vi "Configure Channels.vi"(8 "error in":errorcluster, 11 "HDO4000A Base CFG in":refnum<class "HDO4000A Base CFG.lvclass">) -> (0 "error out":errorcluster, 3 "HDO4000A Base CFG out":refnum<class "HDO4000A Base CFG.lvclass">)   [LabVIEW 2023, in "HDO4000A Base CFG.lvclass"]
uses:
  HDO4000A Base CFG.lvclass
  D:/git/HAL/Configuration Base/Configuration Base.lvclass
  D:/git/HAL/Scope VISA/Configuration/Scope VISA CFG.lvclass
  HAL/Scope VISA/Configuration/Scope VISA CFG.lvclass/Scope VISA CFG.ctl
  HAL/Configuration Base/Configuration Base.lvclass/Configuration Base.ctl
  1880163a-4361-407a-b3a4-4a21bf3de2cd.vi
  95c443c2-3777-477c-973f-d948cfa8a8a4.vi
  0a1f02e3-89ee-415e-b632-0a5c4b782606.vi
  6b7b7499-5745-4b63-8d29-6fa9ae9ebfc2.vi
  0b9faeda-f93b-43a9-80fc-245254112aa6.vi
  15a4e368-5e2e-4ceb-9445-3dca4af458c7.vi
  f2f44aa7-3266-48fd-b649-b0f434fb3c1c.vi
  aee8a4b4-0c09-4a90-9b34-d1bd9b76e547.vi
  <vilib>/JDP Science/JSONtext/Find Item.vi
  <vilib>/JDP Science/JSONtext/Next JSON Value.vi
  <vilib>/JDP Science/JSONtext/String Subset.vi
  <vilib>/JDP Science/JSONtext/Parsing/Advance past next JSON Value (inlined COPY).vi
  <vilib>/JDP Science/JSONtext/Parsing/Advance past whitespace.vi
  <vilib>/JDP Science/JSONtext/Parsing/Advance past String.vi
  <vilib>/JDP Science/JSONtext/Parsing/Advance past Number.vi
  <vilib>/JDP Science/JSONtext/Parsing/Advance past Line Ending.vi
  <vilib>/JDP Science/JSONtext/Parsing/Parse Full Path or Item Name.vi
  <vilib>/JDP Science/JSONtext/Parsing/Advance past Array.vi
  <vilib>/JDP Science/JSONtext/Parsing/Advance past Object.vi
  <vilib>/JDP Science/JSONtext/support/Error Cluster From Code.vi
  <vilib>/JDP Science/JSONtext/Offset/Find Item Locations by Path.vi
  <vilib>/JDP Science/JSONtext/JSON text to Variant.vi
  <vilib>/Utility/error.llb/Error Cluster From Error Code.vi
  <vilib>/JDP Science/JSONtext/LVClass Serializer/JSONtext LVClass Serializer.lvclass
  <vilib>/ErrorRing/Error Ring.xnode
  HDO4000A Base CFG.lvclass/HDO4000A Base CFG.ctl
  <instrlib>/LeCroy Wave Series/LeCroy Wave Series.lvlib
  HAL/Scope VISA/Configuration/Scope VISA CFG.lvclass
  HAL/Configuration Base/Configuration Base.lvclass
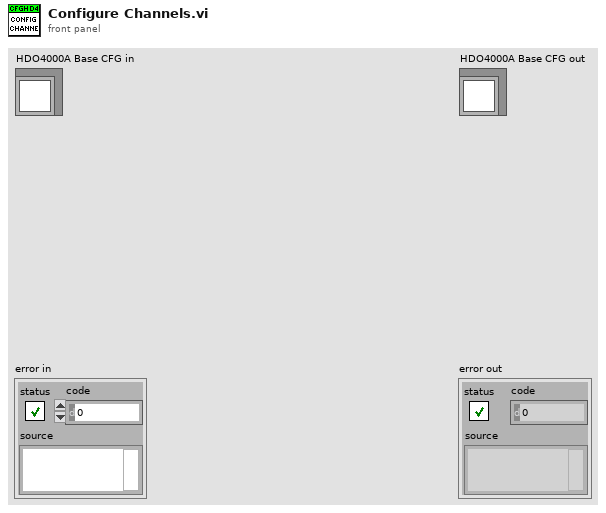
[diagram p1: front panel]
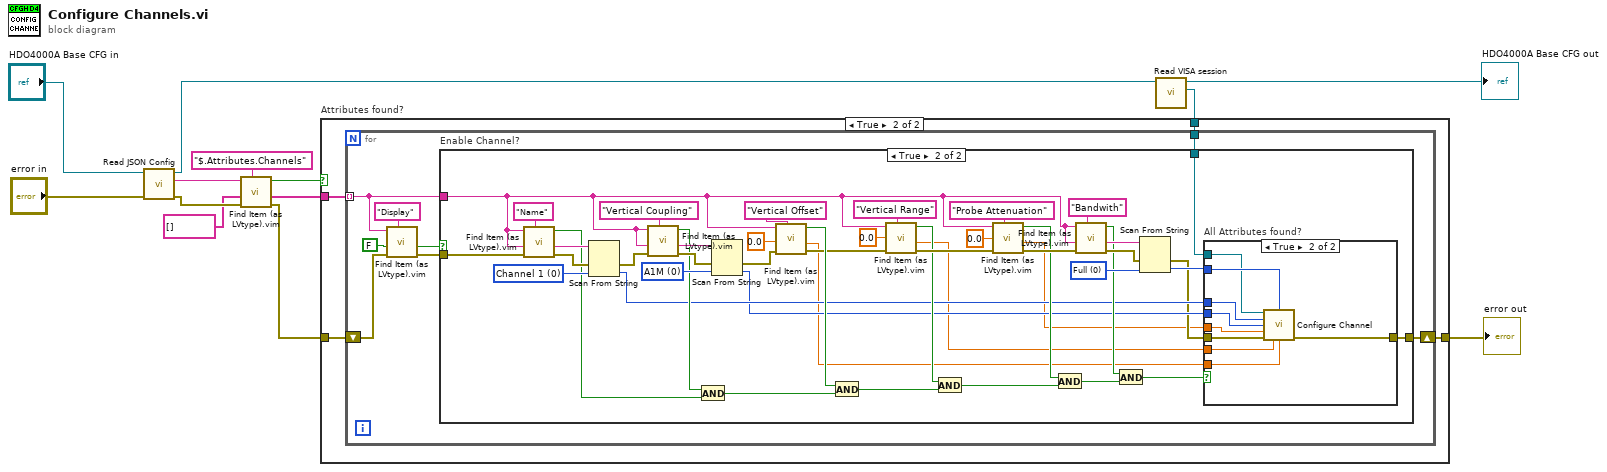
[diagram p0: block diagram]
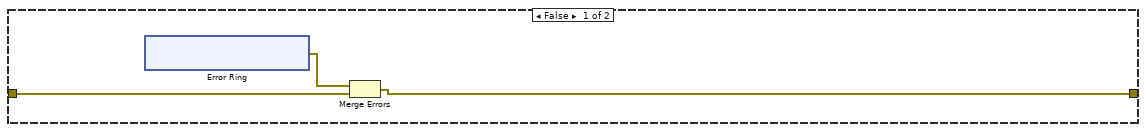
[diagram p2: hidden frame]
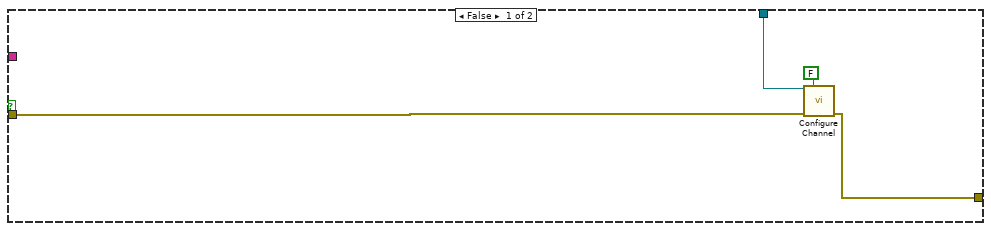
[diagram p3: hidden frame]
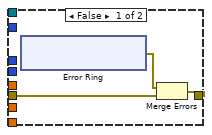
[diagram p4: hidden frame]
diagram:
  n1 = call "Read JSON Config.vi"("error in (no error)"="error in", "object in"="HDO4000A Base CFG in") -> ("error out"=w11:errorcluster, "<JSON>Config"=w8:string, "object out"=w9:refnum<class "HDO4000A Base CFG.lvclass">)  [unwired: 7 in]
  n2 = call "Find Item (as LVtype).vim"("$Path or Item Name"="$.Attributes.Channels", "error in (no error)"=w11, "Data Type and Default Value"=string[] [], "JSON"=w8) -> ("error out"=w4:errorcluster, "Data"=w5:string[], "Found"=w3:bool)  [unwired: 4 in, 1 out]
  n3 = call "Read VISA session.vi"("Scope VISA CFG in"=w9) -> ("VISA session"=w2:refnum<visa-resource-name>, "Scope VISA CFG out"=→"HDO4000A Base CFG out":refnum<class "HDO4000A Base CFG.lvclass">)  [unwired: 8 in, 1 out]
  n4 = case "Attributes found?" shown="True" w3 {
    tunnel: w5 -> [_ w25]
    tunnel: w4 -> [w16 w23]
    tunnel: w2 -> [_ w24]
    tunnel: [w14 w22] -> w1
    frame False {
      n5 = xnode "Error Ring"() -> ("error out"=w15:errorcluster)
      n6 = Merge Errors(w15, w16) -> (w14:errorcluster)
    }
    frame True {
      n7 = for {
        tunnel: w25 -> [w32] mode=indexing
        tunnel: w24 -> [w28]
        shift-right: [w27] -> w22
        shift-left: w23 -> [w26]
        n8 = call "Find Item (as LVtype).vim"("$Path or Item Name"="Display", "error in (no error)"=w26, "Data Type and Default Value"=FALSE, "JSON"=w32) -> ("error out"=w29:errorcluster, "Data"=w33:bool)  [unwired: 4 in, 2 out]
        n9 = case "Enable Channel?" shown="True" w33 {
          tunnel: w32 -> [_ w58]
          tunnel: w29 -> [w35 w82]
          tunnel: w28 -> [w37 w45]
          tunnel: [w34 w38] -> w27
          frame False {
            n10 = call <instrlib>:"Configure Channel.vi"("VISA resource name"=w37, "Enable Channel (T:On)"=FALSE, "error in (no error)"=w35) -> ("error out"=w34:errorcluster)  [unwired: 11 in, 1 out]
          }
          frame True {
            w54 = u16 0 items=["Full", "20MHZ", "25MHZ", "200MHZ", "250MHZ", "1GHZ", "3GHZ", "4GHZ"] ("Bandwidth (0: Full)")
            w75 = u16 0 items=["Channel 1", "Channel 2", "Channel 3", "Channel 4", "Channel 5", "Channel 6", "Channel 7", "Channel 8"] ("Channel (0: Channel 1)")
            w74 = u16 0 items=["A1M", "D1M", "D50", "Ground", "DC", "AC"] ("Vertical Coupling (0: A1M)")
            n11 = call "Find Item (as LVtype).vim"("$Path or Item Name"="Name", "error in (no error)"=w82, "Data Type and Default Value"=w58, "JSON"=w58) -> ("error out"=w79:errorcluster, "Data"=w80:string, "Found"=w71:bool)  [unwired: 4 in, 1 out]
            n12 = Scan From String(input string=w80, error in=w79, default 1=w75) -> (error out=w66:errorcluster, output 1=w44:u16)  [unwired: 2 in, 2 out]
            n13 = call "Find Item (as LVtype).vim"("$Path or Item Name"="Vertical Coupling", "error in (no error)"=w66, "Data Type and Default Value"=w58, "JSON"=w58) -> ("error out"=w78:errorcluster, "Data"=w77:string, "Found"=w70:bool)  [unwired: 4 in, 1 out]
            n14 = And(x=w70, y=w71) -> (x .and. y?=w69:bool)
            n15 = Scan From String(input string=w77, error in=w78, default 1=w74) -> (error out=w67:errorcluster, output 1=w43:u16)  [unwired: 2 in, 2 out]
            n16 = call "Find Item (as LVtype).vim"("$Path or Item Name"="Vertical Offset", "error in (no error)"=w67, "Data Type and Default Value"=0.0, "JSON"=w58) -> ("error out"=w63:errorcluster, "Data"=w40:dbl, "Found"=w68:bool)  [unwired: 4 in, 1 out]
            n17 = And(x=w68, y=w69) -> (x .and. y?=w53:bool)
            n18 = call "Find Item (as LVtype).vim"("$Path or Item Name"="Vertical Range", "error in (no error)"=w63, "Data Type and Default Value"=0.0, "JSON"=w58) -> ("error out"=w60:errorcluster, "Data"=w41:dbl, "Found"=w52:bool)  [unwired: 4 in, 1 out]
            n19 = And(x=w52, y=w53) -> (x .and. y?=w50:bool)
            n20 = call "Find Item (as LVtype).vim"("$Path or Item Name"="Probe Attenuation", "error in (no error)"=w60, "Data Type and Default Value"=0.0, "JSON"=w58) -> ("error out"=w57:errorcluster, "Data"=w39:dbl, "Found"=w51:bool)  [unwired: 4 in, 1 out]
            n21 = And(x=w51, y=w50) -> (x .and. y?=w47:bool)
            n22 = call "Find Item (as LVtype).vim"("$Path or Item Name"="Bandwith", "error in (no error)"=w57, "Data Type and Default Value"=w58, "JSON"=w58) -> ("error out"=w55:errorcluster, "Data"=w56:string, "Found"=w48:bool)  [unwired: 4 in, 1 out]
            n23 = And(x=w48, y=w47) -> (x .and. y?=w46:bool)
            n24 = Scan From String(input string=w56, error in=w55, default 1=w54) -> (error out=w42:errorcluster, output 1=w49:u16)  [unwired: 2 in, 2 out]
            n25 = case "All Attributes found?" shown="True" w46 {
              tunnel: w49 -> [_ w99]
              tunnel: w45 -> [_ w98]
              tunnel: w44 -> [_ w97]
              tunnel: w43 -> [_ w96]
              tunnel: w39 -> [_ w95]
              tunnel: w41 -> [_ w94]
              tunnel: w40 -> [_ w93]
              tunnel: w42 -> [w84 w92]
              tunnel: [w83 w91] -> w38
              frame False {
                n26 = xnode "Error Ring"() -> ("error out"=w85:errorcluster)
                n27 = Merge Errors(w85, w84) -> (w83:errorcluster)
              }
              frame True {
                n28 = call <instrlib>:"Configure Channel.vi"("VISA resource name"=w98, "Bandwidth (0: Full)"=w99, "Channel (0: Channel 1)"=w97, "Vertical Coupling (0: A1M)"=w96, "Probe Attenuation (-1.0)"=w95, "error in (no error)"=w92, "Vertical Range (10.0 V)"=w94, "Vertical Offset (0.0 V)"=w93) -> ("error out"=w91:errorcluster)  [unwired: 6 in, 1 out]
              }
            }
          }
        }
      }
    }
  }
  "error out" <- w1
